vi "RTS Write Config Key.vi"(6 "Chamber 1-1":T1 {"Start Time" format="%<%X\n%x>T"; "End Time" format="%<%X\n%x>T"}, 7 "Loop Index":i32, 8 "error in (no error)":errorcluster, 9 "Relay Name (Freezer, Cab,Slide)":string, 11 "Refnum in":T4) -> (0 "error out":errorcluster, 3 "Refnum out":T4)   [LabVIEW 2020]
uses:
  <vilib>/Utility/config.llb/Config Data RefNum.ctl
  Type Definitions/RTS Door Ops Client.ctl
  Type Definitions/RTS Door Opening Schedule.ctl
  Type Definitions/RTS Door Ops Sequence.ctl
  <vilib>/Utility/config.llb/Write Key (Double).vi
  <vilib>/Utility/config.llb/Write Key (Boolean).vi
  <vilib>/Utility/config.llb/Write Key (I32).vi
  <vilib>/Utility/config.llb/NI_LVConfig.lvlib
panel:
  # "Chamber Conditions:"
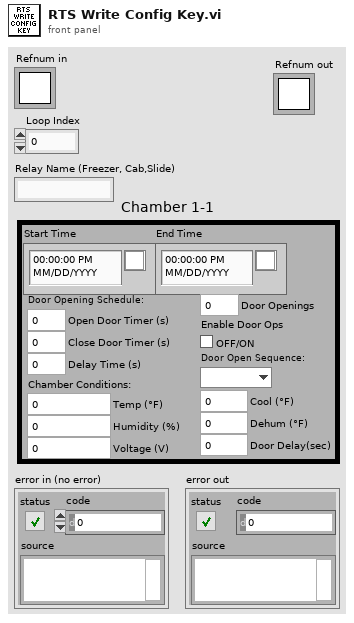
[diagram p1: front panel]
types:
  T1 = typedef "RTS Door Ops Client.ctl" = cluster{"End Time":timestamp, "Start Time":timestamp, "Door Opening Schedule:":T2, "Enable Door Ops":bool, "Door Openings":u32, "Temp (°F)":dbl, "Humidity (%)":dbl, "Voltage (V)":dbl, "Door Open Sequence:":T3, "Door Delay(sec)":dbl, "Dehum (°F)":dbl, "Cool (°F)":dbl}
  T2 = typedef "RTS Door Opening Schedule.ctl" = cluster{"Open Door Timer (s)":dbl, "Delay Time (s)":dbl, "Close Door Timer (s)":dbl}
  T3 = typedef "RTS Door Ops Sequence.ctl" = enum16{"", "1st", "2nd", "3rd"}
  T4 = typedef "NI_LVConfig.lvlib/Config Data RefNum.ctl" = refnum<k1>
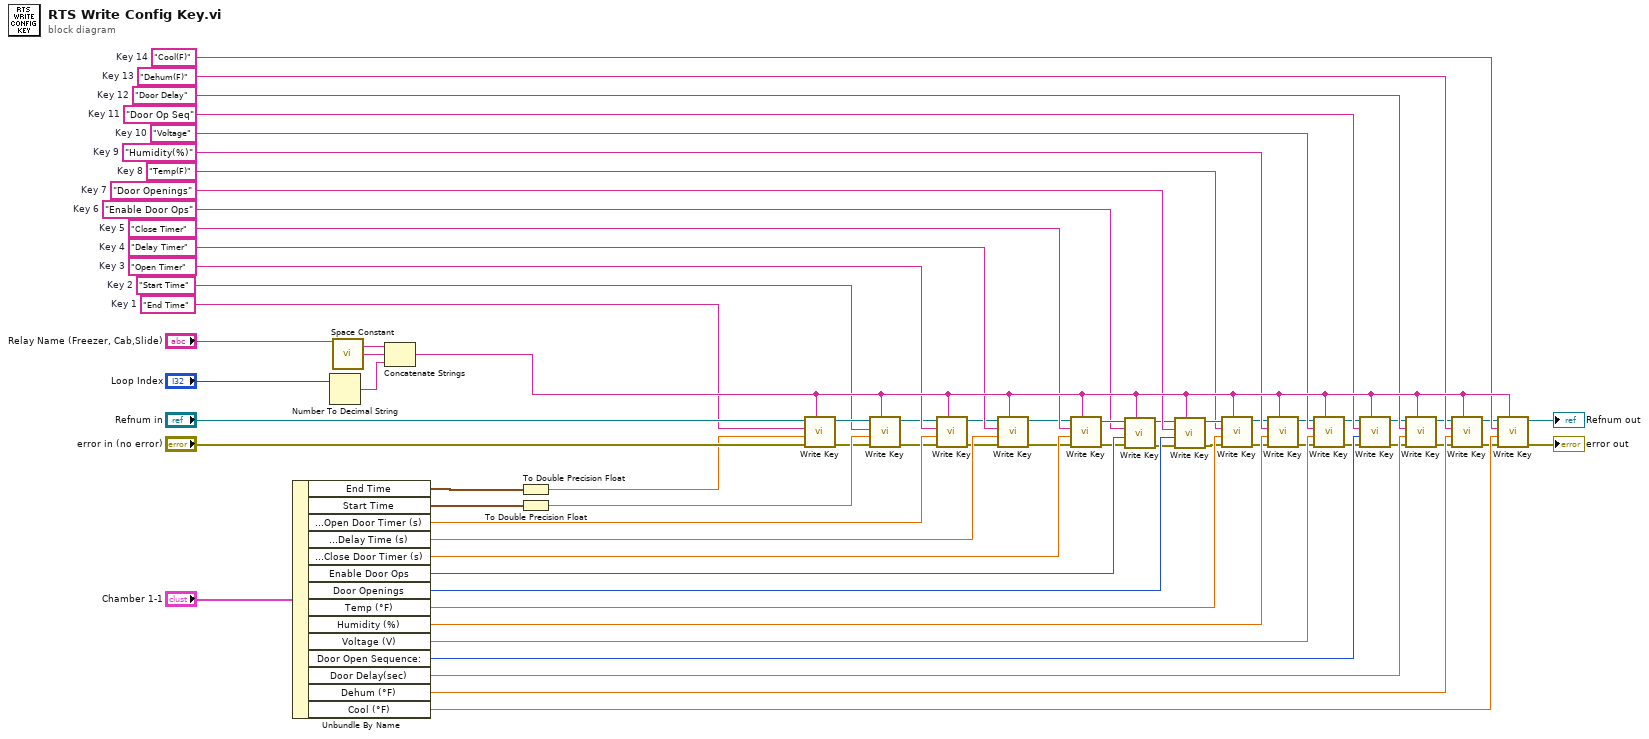
[diagram p0: block diagram]
diagram:
  w23 = "Cool(F)"  # Key 14
  w22 = "Dehum(F)"  # Key 13
  w21 = "Door Delay"  # Key 12
  w20 = "Door Op Seq"  # Key 11
  w19 = "Voltage"  # Key 10
  w18 = "Humidity(%)"  # Key 9
  w17 = "Temp(F)"  # Key 8
  w52 = "Door Openings"  # Key 7
  w43 = "Enable Door Ops"  # Key 6
  w40 = "Close Timer"  # Key 5
  w39 = "Delay Timer"  # Key 4
  w32 = "Open Timer"  # Key 3
  w2 = "Start Time"  # Key 2
  w27 = "End Time"  # Key 1
  n1 = Unbundle By Name("Chamber 1-1") -> ("End Time"=w24:timestamp, "Start Time"=w29:timestamp, "Door Opening Schedule:.Open Door Timer (s)"=w34:dbl, "Door Opening Schedule:.Delay Time (s)"=w41:dbl, "Door Opening Schedule:.Close Door Timer (s)"=w42:dbl, "Enable Door Ops"=w46:bool, "Door Openings"=w51:u32, "Temp (°F)"=w53:dbl, "Humidity (%)"=w54:dbl, "Voltage (V)"=w55:dbl, "Door Open Sequence:"=w56:T3, "Door Delay(sec)"=w57:dbl, "Dehum (°F)"=w58:dbl, "Cool (°F)"=w59:dbl)
  n2 = Number To Decimal String(number="Loop Index") -> (decimal integer string=w61:string)  [unwired: 1 in]
  n3 = call <vilib>:"Space Constant.vi"() -> ("String"=w62:string)
  n4 = Concatenate Strings("Relay Name (Freezer, Cab,Slide)", w62, w61) -> (w64:string)
  n5 = To Double Precision Float(number=w24) -> (double precision float=w28:dbl)
  n6 = To Double Precision Float(number=w29) -> (double precision float=w30:dbl)
  n7 = call-poly <vilib>:"Write Key.vi"("section"=w64, "error in (no error)"="error in (no error)", "value"=w28, "key"=w27, "refnum"="Refnum in") -> ("error out"=w26:errorcluster, "refnum out"=w25:T4)  [unwired: 3 in, 2 out]
  n8 = call-poly <vilib>:"Write Key.vi"("section"=w64, "error in (no error)"=w26, "value"=w30, "key"=w2, "refnum"=w25) -> ("error out"=w33:errorcluster, "refnum out"=w31:T4)  [unwired: 3 in, 2 out]
  n9 = call-poly <vilib>:"Write Key.vi"("section"=w64, "error in (no error)"=w33, "value"=w34, "key"=w32, "refnum"=w31) -> ("error out"=w35:errorcluster, "refnum out"=w37:T4)  [unwired: 3 in, 2 out]
  n10 = call-poly <vilib>:"Write Key.vi"("section"=w64, "error in (no error)"=w35, "value"=w41, "key"=w39, "refnum"=w37) -> ("error out"=w36:errorcluster, "refnum out"=w38:T4)  [unwired: 3 in, 2 out]
  n11 = call-poly <vilib>:"Write Key.vi"("section"=w64, "error in (no error)"=w36, "value"=w42, "key"=w40, "refnum"=w38) -> ("error out"=w44:errorcluster, "refnum out"=w45:T4)  [unwired: 3 in, 2 out]
  n12 = call-poly <vilib>:"Write Key.vi"("section"=w64, "error in (no error)"=w44, "value"=w46, "key"=w43, "refnum"=w45) -> ("error out"=w49:errorcluster, "refnum out"=w47:T4)  [unwired: 4 in, 1 out]
  n13 = call-poly <vilib>:"Write Key.vi"("section"=w64, "error in (no error)"=w49, "value"=w51, "key"=w52, "refnum"=w47) -> ("error out"=w50:errorcluster, "refnum out"=w48:T4)  [unwired: 3 in, 2 out]
  n14 = call-poly <vilib>:"Write Key.vi"("section"=w64, "error in (no error)"=w50, "value"=w53, "key"=w17, "refnum"=w48) -> ("error out"=w3:errorcluster, "refnum out"=w4:T4)  [unwired: 4 in, 1 out]
  n15 = call-poly <vilib>:"Write Key.vi"("section"=w64, "error in (no error)"=w3, "value"=w54, "key"=w18, "refnum"=w4) -> ("error out"=w10:errorcluster, "refnum out"=w5:T4)  [unwired: 4 in, 1 out]
  n16 = call-poly <vilib>:"Write Key.vi"("section"=w64, "error in (no error)"=w10, "value"=w55, "key"=w19, "refnum"=w5) -> ("error out"=w11:errorcluster, "refnum out"=w6:T4)  [unwired: 4 in, 1 out]
  n17 = call-poly <vilib>:"Write Key.vi"("section"=w64, "error in (no error)"=w11, "value"=w56, "key"=w20, "refnum"=w6) -> ("error out"=w12:errorcluster, "refnum out"=w7:T4)  [unwired: 4 in, 1 out]
  n18 = call-poly <vilib>:"Write Key.vi"("section"=w64, "error in (no error)"=w12, "value"=w57, "key"=w21, "refnum"=w7) -> ("error out"=w13:errorcluster, "refnum out"=w8:T4)  [unwired: 4 in, 1 out]
  n19 = call-poly <vilib>:"Write Key.vi"("section"=w64, "error in (no error)"=w13, "value"=w58, "key"=w22, "refnum"=w8) -> ("error out"=w14:errorcluster, "refnum out"=w9:T4)  [unwired: 4 in, 1 out]
  n20 = call-poly <vilib>:"Write Key.vi"("section"=w64, "error in (no error)"=w14, "value"=w59, "key"=w23, "refnum"=w9) -> ("error out"=→"error out":errorcluster, "refnum out"=→"Refnum out":T4)  [unwired: 4 in, 1 out]
